vi "Enter.vi"(8 "error in (no error)":errorcluster, 11 "Door":refnum<class "Door.lvclass">) -> (0 "error out":errorcluster, 3 "Door":refnum<class "Door.lvclass">)   [LabVIEW 2020, in "Door.lvclass"]
uses:
  Door.lvclass
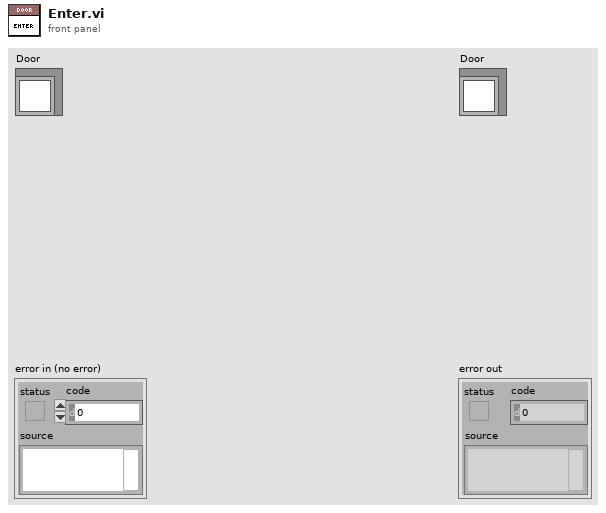
[diagram p1: front panel]
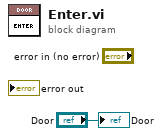
[diagram p0: block diagram]
diagram:
  "Door" <- "Door"
